vi "GrosorCajas.vi"(0 "Imagen":T1(plugin-control), 5 "x_min":i32, 7 "y_min":i32, 9 "x_max":i32, 11 "y_max":i32, 12 "Color":u32(colorbox)=1244928, 13 "Grosor":i32) -> (4 "Imagen salida":T1(plugin-control))   [LabVIEW 2025]
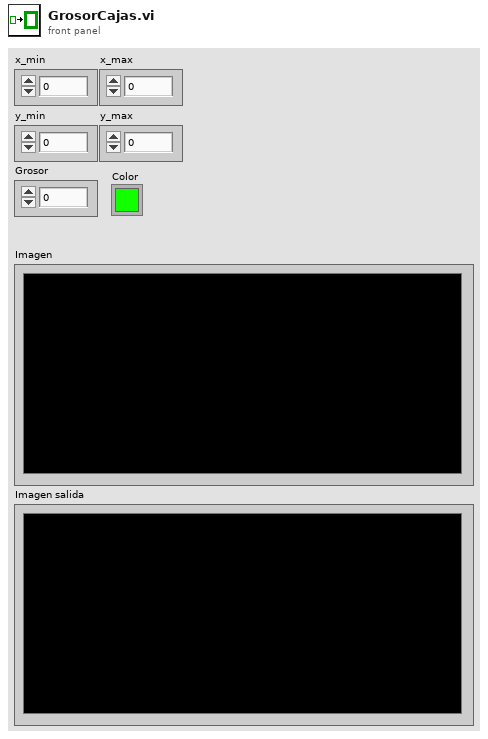
[diagram p1: front panel]
types:
  T1 = typedef "IMAQ Image.ctl" = refnum<image>
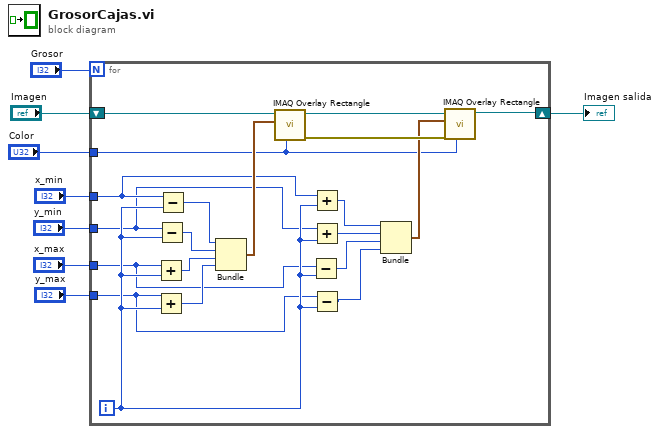
[diagram p0: block diagram]
diagram:
  n1 = for {
    N: "Grosor" -> [_]
    tunnel: "x_min" -> [w21]
    tunnel: "y_min" -> [w20]
    tunnel: "x_max" -> [w19]
    tunnel: "y_max" -> [w18]
    shift-right: [w10] -> w2
    shift-left: "Imagen" -> [w28]
    tunnel: "Color" -> [w9]
    i -> [w22]
    n2 = Add(x=w19, y=w22) -> (x+y=w25:i32)
    n3 = Add(x=w18, y=w22) -> (x+y=w24:i32)
    n4 = Subtract(x=w20, y=w22) -> (x-y=w26:i32)
    n5 = Subtract(x=w21, y=w22) -> (x-y=w27:i32)
    n6 = Bundle(w27, w26, w25, w24) -> (w23:cluster{i32, i32, i32, i32})  [unwired: 1 in]
    n7 = call "IMAQ Overlay Rectangle"("Color"=w9, "Rectangle"=w23, "Image"=w28) -> ("error out"=w12:errorcluster, "Image Out"=w13:T1)  [unwired: 7 in]
    n8 = Subtract(x=w19, y=w22) -> (x-y=w15:i32)
    n9 = Add(x=w21, y=w22) -> (x+y=w17:i32)
    n10 = Add(x=w20, y=w22) -> (x+y=w16:i32)
    n11 = Subtract(x=w18, y=w22) -> (x-y=w14:i32)
    n12 = Bundle(w17, w16, w15, w14) -> (w11:cluster{i32, i32, i32, i32})  [unwired: 1 in]
    n13 = call "IMAQ Overlay Rectangle"("Color"=w9, "error in (no error)"=w12, "Rectangle"=w11, "Image"=w13) -> ("Image Out"=w10:T1)  [unwired: 6 in, 1 out]
  }
  "Imagen salida" <- w2
